vi "GetGroupPhasors.vi"(8 "error in (no error)":errorcluster, 10 "waveforms":waveform(sgl)[](array[waveform]), 11 "Group in":T1) -> (0 "error out":errorcluster, 3 "Group out":T1)   [LabVIEW 2017, in "McsaAnalysisLowRate.lvlib"]
uses:
  <vilib>/addons/InsightCM/Devices/Shared/Mcsa/McsaAnalysisLowRate/McsaAnalysisLowRate.lvlib
  <vilib>/addons/InsightCM/Devices/Shared/Mcsa/McsaAnalysisLowRate/controls/Group.ctl
  <vilib>/addons/InsightCM/Utilities/Analysis/MCSA/controls/McsaChannel.ctl
  <vilib>/addons/InsightCM/Utilities/Analysis/Shared/controls/Feature.ctl
  <vilib>/addons/InsightCM/Utilities/Analysis/Shared/controls/AmplitudeScale.ctl
  <vilib>/addons/InsightCM/MessageBus/Base/controls/KeyValuePair.ctl
  <vilib>/addons/InsightCM/Utilities/Analysis/MCSA/controls/McsaChannelPhasor.ctl
  <vilib>/addons/InsightCM/Utilities/Analysis/MCSA/controls/McsaMotor.ctl
  <vilib>/addons/InsightCM/Utilities/Analysis/MCSA/controls/MotorCalculationCache.ctl
  <vilib>/addons/Electrical Power/Basic/Measurement/subVIs/basic_Power Value.ctl
  <vilib>/addons/InsightCM/Utilities/Analysis/MCSA/controls/TorqueLoadEfficiency.ctl
  <vilib>/addons/InsightCM/Utilities/Analysis/MCSA/McsaAnalysisFunctions.lvlib
  <vilib>/addons/InsightCM/Utilities/MCSA/McsaUtilities.lvlib
  <vilib>/addons/InsightCM/Utilities/Analysis/Shared/AnalysisHelper.lvlib
  <vilib>/addons/Electrical Power/Basic/NI_EP_Basic.lvlib
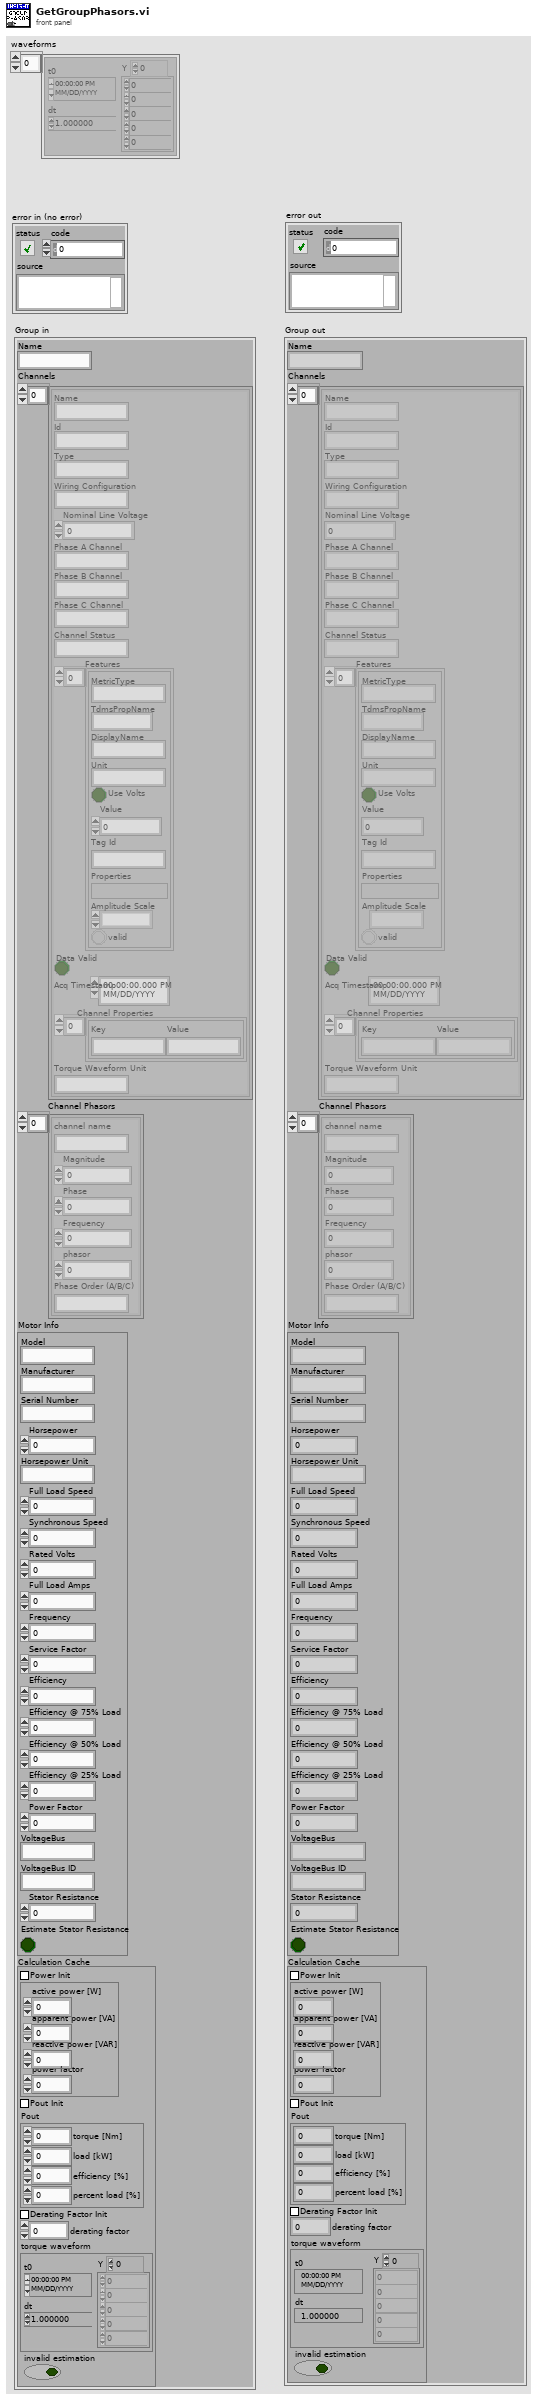
[diagram p1: front panel]
types:
  T1 = typedef "McsaAnalysisLowRate.lvlib/Group.ctl" = cluster{"Name":string, "Channels":T2[], "Channel Phasors":T6[], "Motor Info":T7, "Calculation Cache":T8}
  T2 = typedef "McsaAnalysisFunctions.lvlib/McsaChannel.ctl" = cluster{"Name":string, "Id":string, "Type":string, "Wiring Configuration":string, "Nominal Line Voltage":dbl, "Phase A Channel":string, "Phase B Channel":string, "Phase C Channel":string, "Channel Status":string, "Features":T3[], "Data Valid":bool, "Acq Timestamp":timestamp, "Channel Properties":T5[], "Torque Waveform Unit":string}
  T3 = typedef "AnalysisHelper.lvlib/Feature.ctl" = cluster{"MetricType":string, "TdmsPropName":string, "DisplayName":string, "Unit":string, "Use Volts":bool, "Value":dbl, "Tag Id":string, "Properties":variant, "Amplitude Scale":T4, "valid":bool}
  T4 = typedef "AnalysisHelper.lvlib/AmplitudeScale.ctl" = enum16{"rms", "peak", "pk-pk"}
  T5 = typedef "KeyValuePair.ctl" = cluster{"Key":string, "Value":string}
  T6 = typedef "McsaAnalysisFunctions.lvlib/McsaChannelPhasor.ctl" = cluster{"channel name":string, "Magnitude":dbl, "Phase":dbl, "Frequency":dbl, "phasor":cdb, "Phase Order (A/B/C)":string}
  T7 = typedef "McsaAnalysisFunctions.lvlib/McsaMotor.ctl" = cluster{"Model":string, "Manufacturer":string, "Serial Number":string, "Horsepower":dbl, "Horsepower Unit":string, "Full Load Speed":dbl, "Synchronous Speed":dbl, "Rated Volts":dbl, "Full Load Amps":dbl, "Frequency":dbl, "Service Factor":dbl, "Efficiency":dbl, "Efficiency @ 75% Load":dbl, "Efficiency @ 50% Load":dbl, "Efficiency @ 25% Load":dbl, "Power Factor":dbl, "VoltageBus":string, "VoltageBus ID":string, "Stator Resistance":dbl, "Estimate Stator Resistance":bool}
  T8 = typedef "McsaAnalysisFunctions.lvlib/MotorCalculationCache.ctl" = cluster{"Power Init":bool, "power value":T9, "Pout Init":bool, "Pout":T10, "Derating Factor Init":bool, "derating factor":sgl, "torque waveform":waveform(dbl), "invalid estimation":bool}
  T9 = typedef "NI_EP_Basic.lvlib/basic_Power Value.ctl" = cluster{"active power [W]":dbl, "apparent power [VA]":dbl, "reactive power [VAR]":dbl, "power factor":dbl}
  T10 = typedef "McsaAnalysisFunctions.lvlib/TorqueLoadEfficiency.ctl" = cluster{"torque [Nm]":dbl, "load [kW]":dbl, "efficiency [%]":dbl, "percent load [%]":dbl}
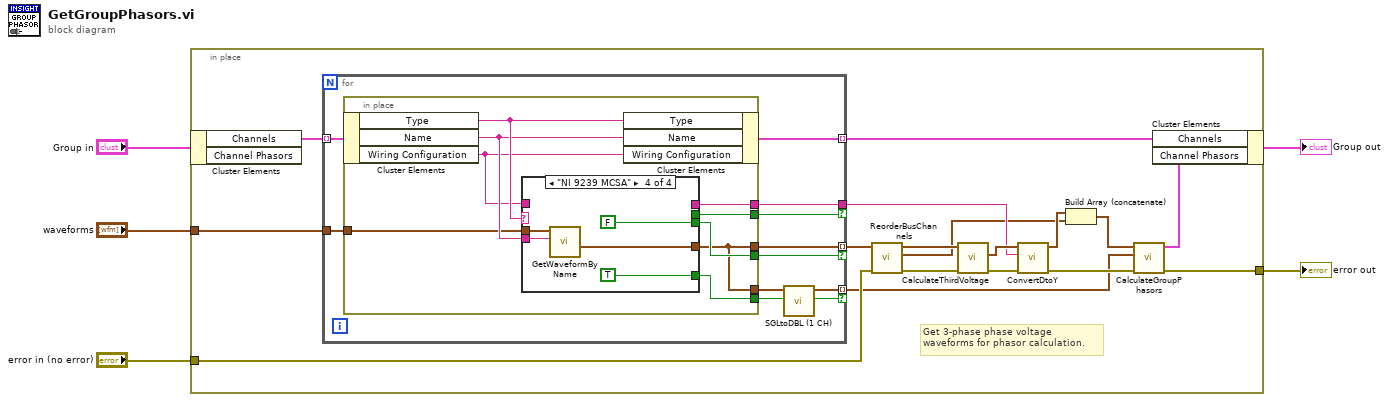
[diagram p0: block diagram]
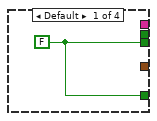
[diagram p2: hidden frame]
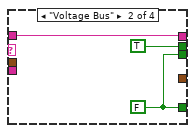
[diagram p3: hidden frame]
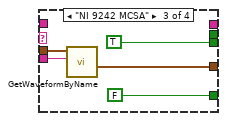
[diagram p4: hidden frame]
diagram:
  n1 = in-place {
    in-place-border: "waveforms" -> [w22]
    in-place-border: "error in (no error)" -> [w11]
    in-place-border: [w21] -> w3
    # "Get 3-phase phase voltage \nwaveforms for phasor calculation."
    n2 = in-place-cluster #1("Group in") -> ("Channels"=w20:T2[])  [unwired: 1 out]
    n3 = for {
      tunnel: w20 -> [w30] mode=indexing
      tunnel: [w32] -> w19 mode=indexing
      tunnel: w22 -> [w31]
      tunnel: [w29] -> w12 mode=indexing if=w28
      tunnel: [w23] -> w6 mode=indexing if=w26
      tunnel: [w25] -> w14 if=w24
      n4 = in-place {
        in-place-border: w31 -> [w39]
        in-place-border: [w37] -> w29
        in-place-border: [w38] -> w28
        in-place-border: [w37] -> w27
        in-place-border: [w36] -> w26
        in-place-border: [w34] -> w25
        in-place-border: [w33] -> w24
        n5 = in-place-cluster #2(w30) -> ("Type"=w41:string, "Name"=w40:string, "Wiring Configuration"=w35:string)
        n6 = case shown="\"NI 9239 MCSA\"" w41 {
          tunnel: w40 -> [_ _ w50 w54]
          tunnel: w39 -> [_ _ w49 w55]
          tunnel: [_ _ w48 w53] -> w37
          tunnel: [w42 w45 TRUE FALSE] -> w38
          tunnel: [w42 w45 FALSE TRUE] -> w36
          tunnel: [_ w44 _ _] -> w34
          tunnel: w35 -> [_ w44 _ _]
          tunnel: [_ TRUE _ _] -> w33
          frame Default {
            w42 = FALSE
          }
          frame "Voltage Bus" {
            w45 = FALSE
          }
          frame "NI 9242 MCSA" {
            n7 = call <vilib>:"GetWaveformByName.vi"("Channel Name"=w50, "Acq Waveforms"=w49) -> ("Waveform"=w48:waveform(sgl))  [unwired: 6 in, 3 out]
          }
          frame "NI 9239 MCSA" {
            n8 = call <vilib>:"GetWaveformByName.vi"("Channel Name"=w54, "Acq Waveforms"=w55) -> ("Waveform"=w53:waveform(sgl))  [unwired: 6 in, 3 out]
          }
        }
        n9 = in-place-cluster #2("Type"=w41, "Name"=w40, "Wiring Configuration"=w35) -> (w32:T2)
      }
      n10 = call <vilib>:"SGLtoDBL (1 CH).vi"("Waveform in"=w27) -> ("Waveform out"=w23:waveform(dbl))  [unwired: 10 in]
    }
    n11 = call <vilib>:"ReorderBusChannels.vi"("error in (no error)"=w11, "Acq Waveforms"=w12) -> ("error out"=w13:errorcluster, "Separated Channels"=w8:waveform(dbl)[], "Bus Waveforms"=w10:waveform(dbl)[])  [unwired: 7 in]
    n12 = call <vilib>:"CalculateThirdVoltage.vi"("error out"=w13, "voltage waveforms in"=w10) -> ("error out"=w16:errorcluster, "3-phases voltage waveforms"=w17:waveform(dbl)[])  [unwired: 7 in, 1 out]
    n13 = call <vilib>:"ConvertDtoY.vi"("error in"=w16, "Wiring Configuration"=w14, "voltage waveform"=w17) -> ("error out"=w15:errorcluster, "phase voltage waveform"=w9:waveform(dbl)[])  [unwired: 7 in]
    n14 = Build Array (concatenate)(w9, w8) -> (w7:waveform(dbl)[])
    n15 = call <vilib>:"CalculateGroupPhasors.vi"("error in"=w15, "current waveforms"=w6, "phase voltage waveforms"=w7) -> ("error out"=w21:errorcluster, "Group Voltage Phasors"=w18:T6[])  [unwired: 7 in]
    n16 = in-place-cluster #1("Channels"=w19, "Channel Phasors"=w18) -> (→"Group out":T1)
  }
  "error out" <- w3
